vi "Decimation Channel.vi"(8 "error in (no error)":errorcluster, 11 "Node Ptr":T1 format="%.0x") -> (0 "error out":errorcluster)   [LabVIEW 2015, in "RefMem DMA Custom Device.lvlib"]
uses:
  RefMem DMA Custom Device.lvlib
  Program Files (x86)/National Instruments/LabVIEW 2015/vi.lib/NI Veristand/Custom Device API/Custom Device Item Ref.ctl
  Program Files (x86)/National Instruments/LabVIEW 2015/vi.lib/NI Veristand/Custom Device API/Custom Device API.lvlib
panel:
  in  "Default Value":dbl min=0.0 step=1.0
  in  "Warning text":string="WARNING: The address selected by this channel is within the range of addresses reserved by NI VeriStand's built in reflective memory support!"
  out "Warn Icon":bool
  in  "Header":cluster{"Section Name":string}={"Section Name"="Data Channel"}
  in  "Description":string="Decimation channel for this block\n0 - disable the block\n1.. set decimation"
  in  "Name":string
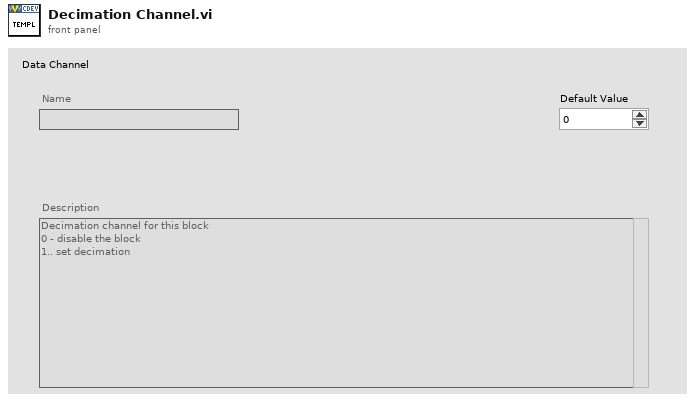
[diagram p1: front panel]
types:
  T1 = typedef "Custom Device API.lvlib/Custom Device Item Ref.ctl" = u64
  T2 = typedef "Custom Device API.lvlib/Custom Device Channel.ctl" = cluster{"Type":T3, "Units":string, "Default Value":dbl, "Faultable":bool, "Scalable":bool}
  T3 = typedef "Custom Device API.lvlib/Custom Device Channel Type.ctl" = enum16{"Input", "Output"}
  T4 = typedef "Custom Device API.lvlib/Custom Device Commands.ctl" = enum16{"Default", "Item renamed", "Shutdown", "Dynamic button pressed"}
  T5 = typedef "Custom Device API.lvlib/Custom Device Item Info.ctl" = cluster{"Name":string, "Is Channel":bool, "GUID":string, "Is Waveform":bool}
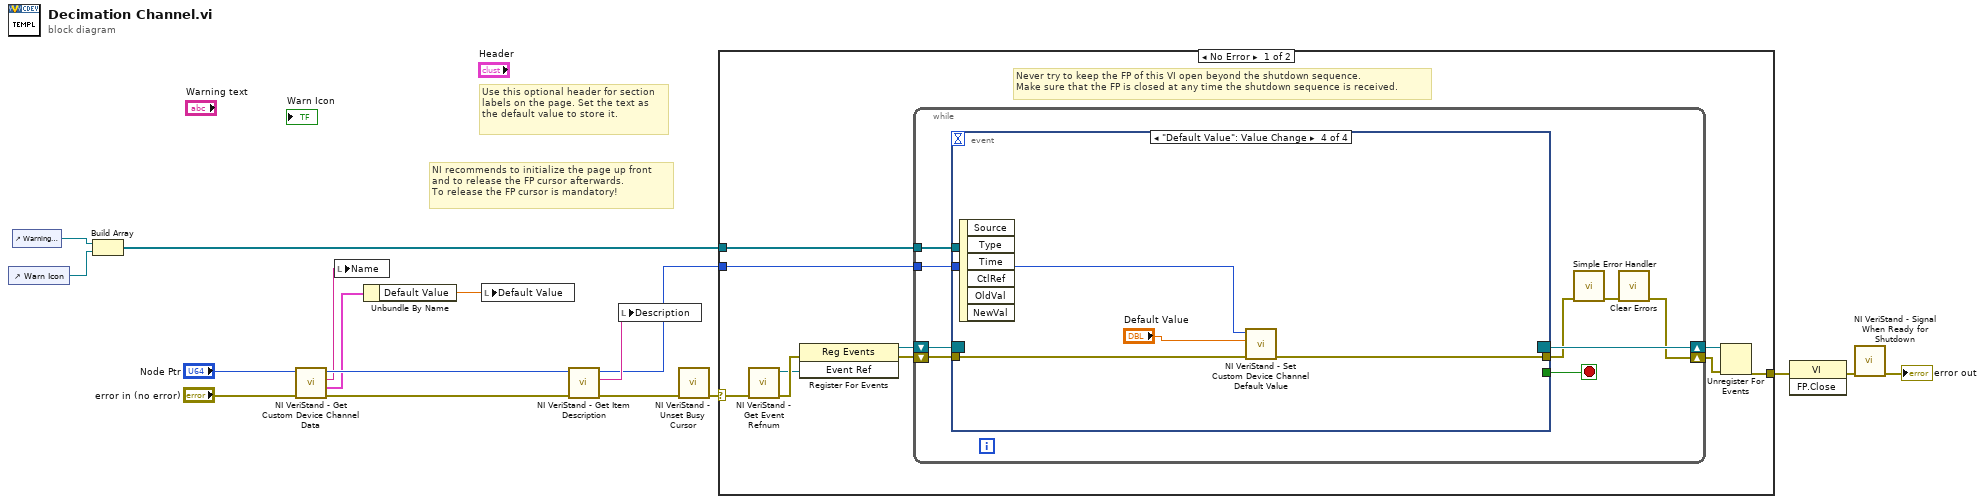
[diagram p0: block diagram]
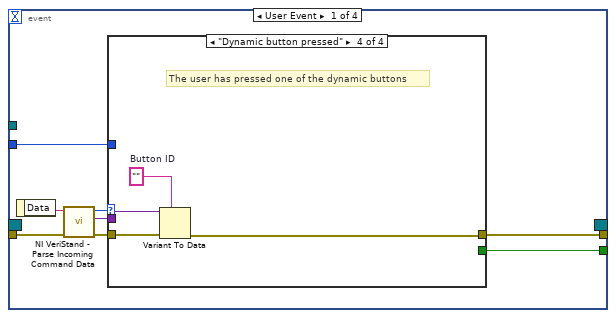
[diagram p2: hidden frame]
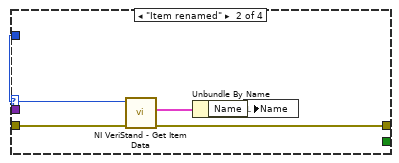
[diagram p4: hidden frame]
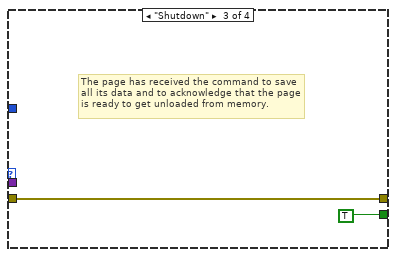
[diagram p5: hidden frame]
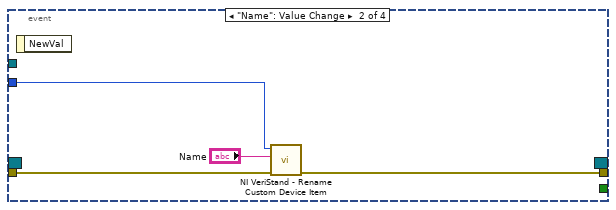
[diagram p6: hidden frame]
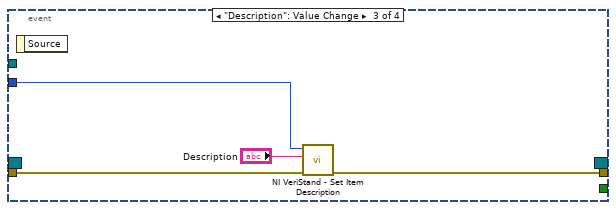
[diagram p7: hidden frame]
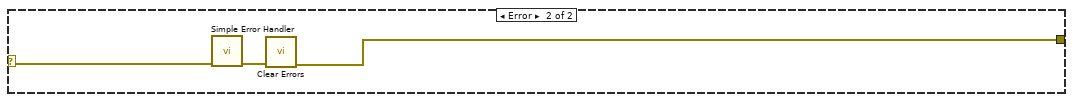
[diagram p8: hidden frame]
diagram:
  # "Use this optional header for section labels on the page. Set the text as the default value to store it."
  # "NI recommends to initialize the page up front\nand to release the FP cursor afterwards.\nTo release the FP cursor is mandatory!"
  n1 = control-ref of="Warn Icon"() -> (w12:refnum<vi>)
  n2 = control-ref of="Warning text"() -> (w11:refnum<vi>)
  n3 = Build Array(w11, w12) -> (w10:refnum<vi>[])
  n4 = call "NI VeriStand - Get Custom Device Channel Data.vi"("error in (no error)"="error in (no error)", "Channel Ref in"="Node Ptr") -> ("error out"=w9:errorcluster, "Channel"=w7:T2, "Channel Name"=w4:string, "Channel Ref out"=w8:T1)  [unwired: 4 in, 2 out]
  n5 = local write "Name"(w4) -> ()
  n6 = Unbundle By Name(w7) -> ("Default Value"=w3:dbl)
  n7 = local write "Default Value"(w3) -> ()
  n8 = call "NI VeriStand - Get Item Description.vi"("error in (no error)"=w9, "Item Ref in"=w8) -> ("error out"=w6:errorcluster, "Description"=w13:string, "Item Ref out"=w5:T1)  [unwired: 7 out]
  n9 = local write "Description"(w13) -> ()
  n10 = call "NI VeriStand - Unset Busy Cursor.vi"("error in (no error)"=w6) -> ("error out"=w14:errorcluster)  [unwired: 10 out]
  n11 = case shown="No Error" w14 {
    selector: w14 -> [w19 w71]
    tunnel: [w24 w69] -> w17
    tunnel: w5 -> [w20 _]
    tunnel: w10 -> [w18 _]
    frame No Error {
      # "Never try to keep the FP of this VI open beyond the shutdown sequence.\nMake sure that the FP is closed at any time the shutdown sequence is received."
      n12 = call "NI VeriStand - Get Event Refnum.vi"("error in (no error)"=w19) -> ("error out"=w27:errorcluster, "Event Ref"=w23:refnum<user-event>)  [unwired: 9 out]
      n13 = register-events(error in=w27, w23) -> (reference out=w21:refnum<event-registration>, error out=w22:errorcluster)  [unwired: 1 in]
      n14 = while {
        tunnel: w20 -> [w32]
        shift-right: [w29] -> w25
        shift-left: w22 -> [w35]
        shift-right: [w36] -> w26
        shift-left: w21 -> [w34]
        tunnel: w18 -> [w28]
        stop <- w33 stop-if-true
        n15 = event shown="[3] \"Default Value\": Value Change" {
          selector: w34 -> [_ _ _ _]
          dyn-events: [_ _ _ _] -> w36
          timeout: _ -> [_ _ _ _]
          tunnel: w35 -> [w44 w60 w63 w67]
          tunnel: [w40 _ _ _] -> w33
          tunnel: [w39 w59 w62 w66] -> w31
          tunnel: w32 -> [w38 w58 w64 w68]
          tunnel: w28 -> [_ _ _ _]
          event User Event {
            n16 = event-data() -> ("Data"=w43:string)  [unwired: 1 out]
            n17 = call "NI VeriStand - Parse Incoming Command Data.vi"("error in (no error)"=w44, "Incoming data"=w43) -> ("error out"=w42:errorcluster, "Outgoing data"=w37:variant, "Action"=w41:T4)  [unwired: 7 out]
            n18 = case shown="\"Dynamic button pressed\"" w41 {
              tunnel: w42 -> [w45 w50 w51 w56]
              tunnel: [_ _ TRUE _] -> w40
              tunnel: [w45 w47 w51 w53] -> w39
              tunnel: w38 -> [_ w49 _ _]
              tunnel: w37 -> [_ _ _ w55]
              frame "Default", Default {
              }
              frame "Item renamed" {
                n19 = call "NI VeriStand - Get Item Data.vi"("error in (no error)"=w50, "Item Ref in"=w49) -> ("error out"=w47:errorcluster, "Item Info"=w48:T5)  [unwired: 8 out]
                n20 = Unbundle By Name(w48) -> ("Name"=w46:string)
                n21 = local write "Name"(w46) -> ()
              }
              frame "Shutdown" {
                # "The page has received the command to save all its data and to acknowledge that the page is ready to get unloaded from memory."
              }
              frame "Dynamic button pressed" {
                w54 = ""  # Button ID
                # "The user has pressed one of the dynamic buttons"
                n22 = Variant To Data(error in=w56, type=w54, Variant=w55) -> (error out=w53:errorcluster)  [unwired: 1 out]
              }
            }
          }
          event "Name": Value Change {
            n23 = event-data() -> ()  [unwired: 2 out]
            n24 = call "NI VeriStand - Rename Custom Device Item.vi"("error in (no error)"=w60, "New Name"="Name", "Item Ref in"=w58) -> ("error out"=w59:errorcluster)  [unwired: 1 in, 7 out]
          }
          event "Description": Value Change {
            n25 = event-data() -> ()  [unwired: 2 out]
            n26 = call "NI VeriStand - Set Item Description.vi"("error in (no error)"=w63, "Description"="Description", "Item Ref in"=w64) -> ("error out"=w62:errorcluster)  [unwired: 8 out]
          }
          event "Default Value": Value Change {
            n27 = event-data() -> ()  [unwired: 7 out]
            n28 = call "NI VeriStand - Set Custom Device Channel Default Value.vi"("error in (no error)"=w67, "Default Value"="Default Value", "Channel Ref in"=w68) -> ("error out"=w66:errorcluster)  [unwired: 7 in, 1 out]
          }
        }
        n29 = call <vilib>:"Simple Error Handler.vi"("error in (no error)"=w31) -> ("error out"=w30:errorcluster)  [unwired: 1 in, 7 out]
        n30 = call <vilib>:"Clear Errors.vi"("error in (no error)"=w30) -> ("error out"=w29:errorcluster)  [unwired: 1 in, 5 out]
      }
      n31 = Unregister For Events(event registration refnum=w26, error in=w25) -> (error out=w24:errorcluster)
    }
    frame Error {
      n32 = call <vilib>:"Simple Error Handler.vi"("error in (no error)"=w71) -> ("error out"=w70:errorcluster)  [unwired: 1 in, 7 out]
      n33 = call <vilib>:"Clear Errors.vi"("error in (no error)"=w70) -> ("error out"=w69:errorcluster)  [unwired: 1 in, 5 out]
    }
  }
  n34 = invoke class="VI" method="FP.Close"(error in=w17) -> (error out=w16:errorcluster)  [unwired: 2 in, 2 out]
  n35 = call "NI VeriStand - Signal When Ready for Shutdown.vi"("error in (no error)"=w16) -> ("error out"=→"error out":errorcluster)  [unwired: 10 out]
